vi "Actividad04.vi"() -> ()   [LabVIEW 2025]
panel:
  in  "stop":bool
  out "Contador":dbl
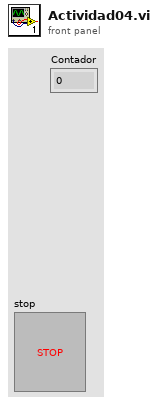
[diagram p1: front panel]
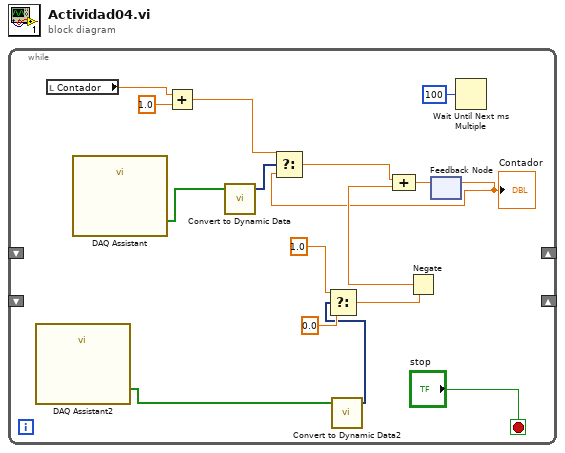
[diagram p0: block diagram]
diagram:
  n1 = while {
    shift-right: _ -> [_]
    shift-left: _ -> [_]
    shift-right: _ -> [_]
    shift-left: _ -> [_]
    stop <- "stop" stop-if-true
    n2 = call "DAQ Assistant2"() -> ("data"=w2:bool[])  [unwired: 17 in, 2 out]
    n3 = local read "Contador"() -> (w8:dbl)
    n4 = call "DAQ Assistant"() -> ("data"=w1:bool[])  [unwired: 17 in, 2 out]
    n5 = Add(x=w8, y=1.0) -> (x+y=w12:dbl)
    n6 = call "Convert to Dynamic Data"("Array"=w1) -> ("Dynamic Data Type"=w4:dynamicdata)  [unwired: 3 in]
    n7 = call "Convert to Dynamic Data2"("Array"=w2) -> ("Dynamic Data Type"=w3:dynamicdata)  [unwired: 3 in]
    n8 = Select(t=1.0, s=w3, f=0.0) -> (s? t:f=w13:dbl)
    n9 = Negate(x=w13) -> (-x=w10:dbl)
    n10 = feedback #1() -> (w6:dbl)  [unwired: 1 in]
    "Contador" <- w6
    n11 = Select(t=w12, s=w4, f=w6) -> (s? t:f=w11:dbl)
    n12 = Compound Arithmetic op=ADD(w11, w10) -> (w7:dbl)
    n13 = feedback-in #1(w7) -> ()
    n14 = Wait Until Next ms Multiple(millisecond multiple=u32 100) -> ()  [unwired: 1 out]
  }
